vi "ProgramControl.vi"(0 "Universal Robot.lvclass in":refnum<class "Universal Robot.lvclass">, 5 "error in (no error)":errorcluster) -> (14 "Universal Robot.lvclass out":refnum<class "Universal Robot.lvclass">, 15 "programReturnStatus":T1, 19 "error out":errorcluster)   [LabVIEW 2016, in "Universal Robot.lvclass"]
uses:
  Universal Robot.lvclass
  ProgramReturnStatus.ctl
  ProgramState.ctl
panel:
  in  "rate":i32=1000
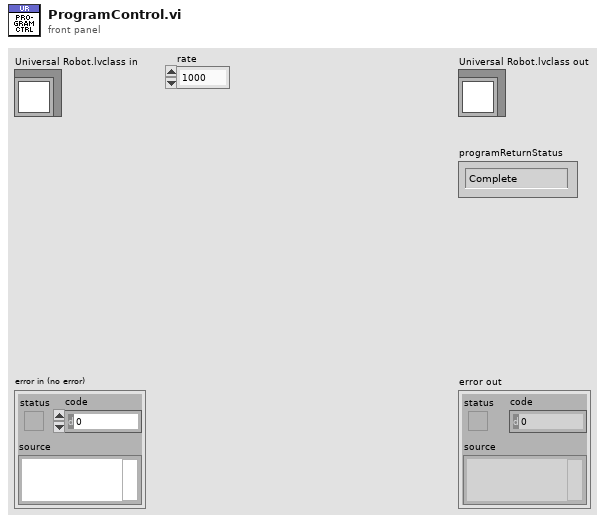
[diagram p1: front panel]
types:
  T1 = typedef "Universal Robot.lvclass/ProgramReturnStatus.ctl" = enum16{"Complete", "Stopped", "Error", "Faulted"}
  T2 = typedef "Universal Robot.lvclass/ProgramState.ctl" = enum16{"STOPPED", "PLAYING", "PAUSE"}
  T3 = typedef "Universal Robot.lvclass/ProgramControlEvent.ctl" = enum16{"Stop", "Pause"}
  T4 = typedef "Universal Robot.lvclass/ProgramStatus.ctl" = cluster{"Loaded Program":string, "Valid Program":bool, "Program State":T2, "Running":bool}
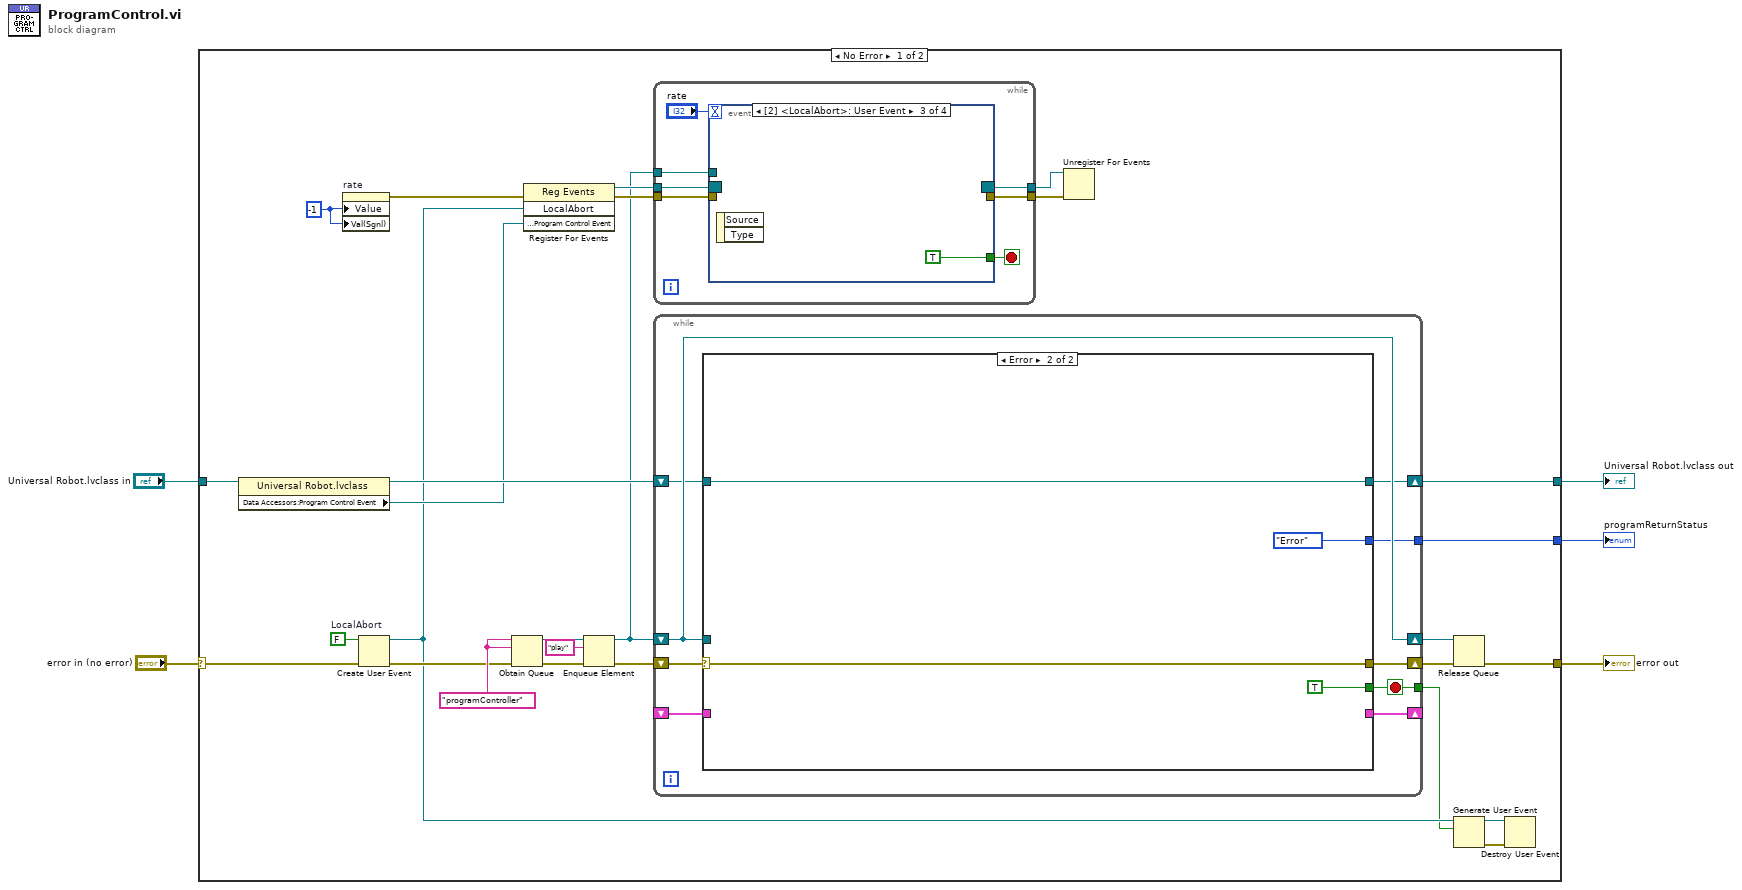
[diagram p0: block diagram]
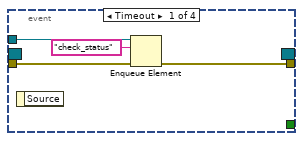
[diagram p2: hidden frame]
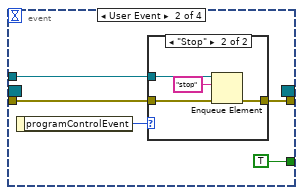
[diagram p3: hidden frame]
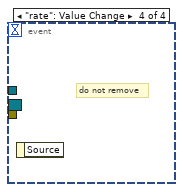
[diagram p5: hidden frame]
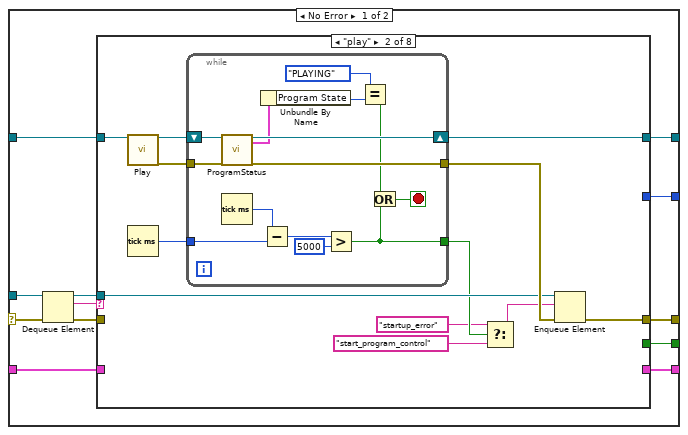
[diagram p6: hidden frame]
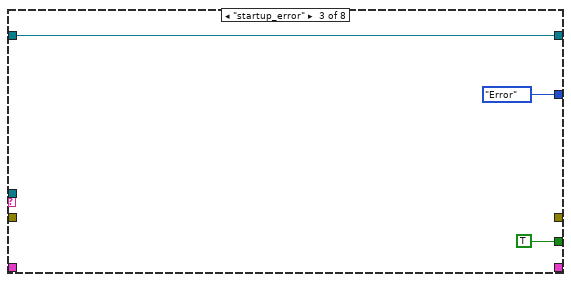
[diagram p8: hidden frame]
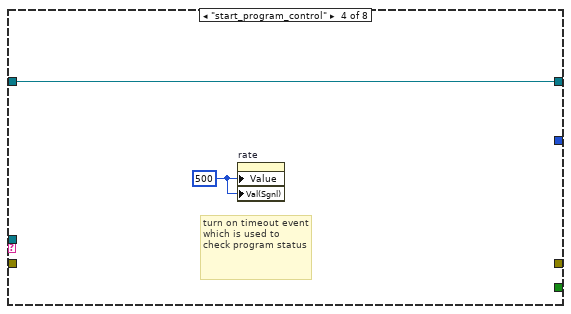
[diagram p9: hidden frame]
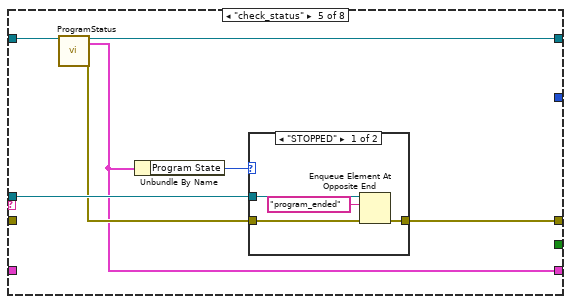
[diagram p10: hidden frame]
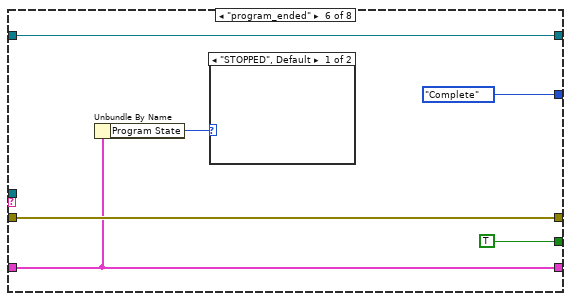
[diagram p12: hidden frame]
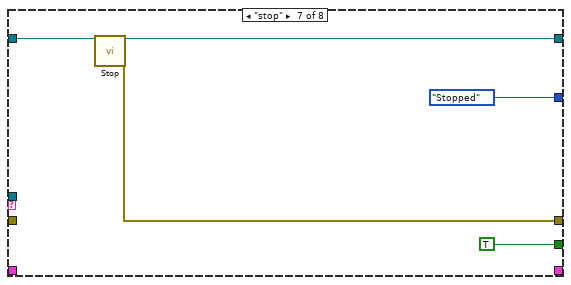
[diagram p14: hidden frame]
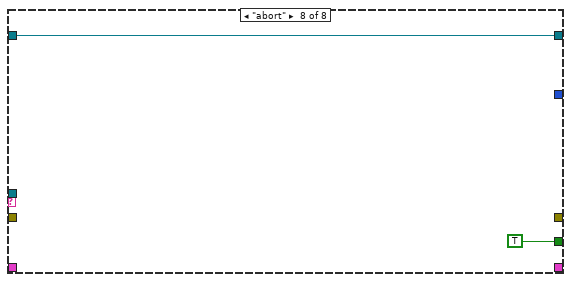
[diagram p15: hidden frame]
diagram:
  n1 = case shown="No Error" "error in (no error)" {
    selector: "error in (no error)" -> [w7 w139]
    tunnel: "Universal Robot.lvclass in" -> [w22 w138]
    tunnel: [w19 _] -> w4
    tunnel: [w9 w139] -> w3
    tunnel: [w8 w138] -> w2
    frame No Error {
      w18 = FALSE  # LocalAbort
      w21 = -1 ("rate")
      w28 = "programController" ("name (unnamed)")
      n2 = property class="Universal Robot.lvclass"(reference=w22) -> (reference out=w27:refnum<class "Universal Robot.lvclass">, "Data Accessors:Program Control Event"=w20:refnum<user-event>)  [unwired: 1 in, 1 out]
      n3 = property on="rate" class="DigNum (strict)"("Value"=w21, "Val(Sgnl)"=w21) -> (error out=w17:errorcluster)  [unwired: 2 in, 1 out]
      n4 = Create User Event(user event datatype=w18, error in=w7) -> (user event=w14:refnum<user-event>, error out=w16:errorcluster)
      n5 = Obtain Queue(name (unnamed)=w28, element data type=w28, error in (no error)=w16) -> (queue out=w26:refnum<queue>, error out=w25:errorcluster)  [unwired: 2 in, 1 out]
      n6 = register-events(error in=w17, w14, w20) -> (reference out=w32:refnum<event-registration>, error out=w31:errorcluster)  [unwired: 1 in]
      n7 = Enqueue Element(queue=w26, element="play", error in (no error)=w25) -> (queue out=w24:refnum<queue>, error out=w23:errorcluster)  [unwired: 1 in, 1 out]
      n8 = while {
        tunnel: w24 -> [w39]
        tunnel: w31 -> [w38]
        tunnel: w32 -> [w37]
        tunnel: [w36] -> w10
        tunnel: [w33] -> w11
        stop <- w35 stop-if-true
        n9 = event shown="[2] <LocalAbort>: User Event" {
          selector: w37 -> [_ _ _ _]
          dyn-events: [_ _ _ _] -> w33
          timeout: "rate" -> [_ _ _ _]
          tunnel: w39 -> [w43 w48 _ _]
          tunnel: w38 -> [w42 w47 _ _]
          tunnel: [w41 w46 _ _] -> w36
          tunnel: [_ TRUE TRUE _] -> w35
          event Timeout {
            n10 = event-data() -> ()  [unwired: 1 in, 1 out]
            n11 = Enqueue Element(queue=w43, element="check_status", error in (no error)=w42) -> (error out=w41:errorcluster)  [unwired: 1 in, 2 out]
          }
          event User Event {
            n12 = event-data() -> ("programControlEvent"=w44:T3)  [unwired: 1 in]
            n13 = case shown="\"Stop\"" w44 {
              tunnel: w48 -> [_ w53]
              tunnel: w47 -> [w49 w52]
              tunnel: [w49 w51] -> w46
              frame Default {
              }
              frame "Stop" {
                n14 = Enqueue Element(queue=w53, element="stop", error in (no error)=w52) -> (error out=w51:errorcluster)  [unwired: 1 in, 2 out]
              }
            }
          }
          event User Event {
            n15 = event-data() -> ()  [unwired: 1 in, 2 out]
          }
          event "rate": Value Change {
            # "do not remove"
            n16 = event-data() -> ()  [unwired: 1 in, 1 out]
          }
        }
      }
      n17 = while {
        shift-right: [w61] -> w30
        shift-left: w23 -> [w63]
        shift-right: [w62] -> w29
        shift-left: w24 -> [w62]
        shift-right: [w59] -> w8
        shift-left: w27 -> [w60]
        shift-right: [w58] -> _
        shift-left: _ -> [w57]
        tunnel: [w56] -> w19
        tunnel: [w55] -> w6
        stop <- w55 stop-if-true
        n18 = case shown="Error" w63 {
          selector: w63 -> [w74 w135]
          tunnel: w62 -> [w75 _]
          tunnel: [w70 w135] -> w61
          tunnel: [w69 TRUE] -> w55
          tunnel: w60 -> [w68 w137]
          tunnel: [w67 w137] -> w59
          tunnel: [w66 _] -> w58
          tunnel: w57 -> [w65 _]
          tunnel: [w64 ProgramReturnStatus."Error" ("programReturnStatus")] -> w56
          frame No Error {
            n19 = Dequeue Element(queue=w75, error in (no error)=w74) -> (queue out=w71:refnum<queue>, element=w72:string, error out=w73:errorcluster)  [unwired: 1 in, 1 out]
            n20 = case shown="\"play\"" w72 {
              tunnel: w73 -> [w77 _ _ _ _ w125 _ _]
              tunnel: w71 -> [_ w82 _ _ w113 _ _ _]
              tunnel: [w77 w84 _ _ w111 w125 w127 _] -> w70
              tunnel: [_ _ TRUE _ _ TRUE TRUE TRUE] -> w69
              tunnel: w68 -> [w76 w89 w106 w108 w115 w126 w129 w132]
              tunnel: [w76 w87 w106 w108 w114 w126 w128 w132] -> w67
              tunnel: [_ _ _ _ w110 w123 _ _] -> w66
              tunnel: w65 -> [_ _ _ _ _ w123 _ _]
              tunnel: [_ _ ProgramReturnStatus."Error" ("programReturnStatus") _ _ ProgramReturnStatus."Complete" ("programReturnStatus") ProgramReturnStatus."Stopped" ("programReturnStatus") _] -> w64
              frame Default {
              }
              frame "play" {
                n21 = call-dynamic "Play.vi"("Universal Robot.lvclass in"=w89) -> ("Universal Robot.lvclass out"=w88:refnum<class "Universal Robot.lvclass">, "error out"=w86:errorcluster)  [unwired: 17 in]
                n22 = Tick Count (ms)() -> (millisecond timer value=w85:u32)
                n23 = while {
                  shift-right: [w102] -> w87
                  shift-left: w88 -> [w103]
                  tunnel: w86 -> [w100]
                  tunnel: w85 -> [w98]
                  tunnel: [w97] -> w83
                  tunnel: [w93] -> w81
                  stop <- w94 stop-if-true
                  n24 = call-dynamic "ProgramStatus.vi"("Universal Robot.lvclass in"=w103, "error in (no error)"=w100) -> ("Universal Robot.lvclass out"=w102:refnum<class "Universal Robot.lvclass">, "Program Status"=w101:T4, "error out"=w97:errorcluster)  [unwired: 15 in]
                  n25 = Tick Count (ms)() -> (millisecond timer value=w99:u32)
                  n26 = Unbundle By Name(w101) -> ("Program State"=w92:T2)
                  n27 = Subtract(x=w99, y=w98) -> (x-y=w96:u32)
                  n28 = Greater?(x=w96, y=u32 5000) -> (0:w93:bool)
                  n29 = Equal?(x=ProgramState."PLAYING", y=w92) -> (x = y?=w90:bool)
                  n30 = Or(x=w90, y=w93) -> (x .or. y?=w94:bool)
                }
                n31 = Select(t="startup_error", s=w81, f="start_program_control") -> (s? t:f=w79:string)
                n32 = Enqueue Element(queue=w82, element=w79, error in (no error)=w83) -> (error out=w84:errorcluster)  [unwired: 1 in, 2 out]
              }
              frame "startup_error" {
              }
              frame "start_program_control" {
                w107 = 500 ("rate")
                # "turn on timeout event which is used to check program status"
                n33 = property on="rate" class="DigNum (strict)"("Value"=w107, "Val(Sgnl)"=w107) -> ()  [unwired: 2 in, 2 out]
              }
              frame "check_status" {
                n34 = call-dynamic "ProgramStatus.vi"("Universal Robot.lvclass in"=w115) -> ("Universal Robot.lvclass out"=w114:refnum<class "Universal Robot.lvclass">, "Program Status"=w110:T4, "error out"=w112:errorcluster)  [unwired: 16 in]
                n35 = Unbundle By Name(w110) -> ("Program State"=w109:T2)
                n36 = case shown="\"STOPPED\"" w109 {
                  tunnel: w113 -> [w119 _]
                  tunnel: w112 -> [w118 w120]
                  tunnel: [w117 w120] -> w111
                  frame "STOPPED" {
                    n37 = Enqueue Element At Opposite End(queue=w119, element="program_ended", error in (no error)=w118) -> (error out=w117:errorcluster)  [unwired: 1 in, 2 out]
                  }
                  frame Default {
                  }
                }
              }
              frame "program_ended" {
                n38 = Unbundle By Name(w123) -> ("Program State"=w122:T2)
                n39 = case shown="\"STOPPED\", Default" w122 {
                  frame "STOPPED", Default {
                  }
                  frame "PLAYING" {
                  }
                }
              }
              frame "stop" {
                n40 = call-dynamic "Stop.vi"("Universal Robot.lvclass in"=w129) -> ("Universal Robot.lvclass out"=w128:refnum<class "Universal Robot.lvclass">, "error out"=w127:errorcluster)  [unwired: 17 in]
              }
              frame "abort" {
              }
            }
          }
          frame Error {
          }
        }
      }
      n41 = Unregister For Events(event registration refnum=w11, error in=w10) -> ()  [unwired: 1 out]
      n42 = Release Queue(queue=w29, error in (no error)=w30) -> (error out=w9:errorcluster)  [unwired: 1 in, 2 out]
      n43 = Generate User Event(user event=w14, event data cluster=w6) -> (user event out=w13:refnum<user-event>, error out=w12:errorcluster)  [unwired: 2 in]
      n44 = Destroy User Event(user event=w13, error in=w12) -> ()  [unwired: 1 out]
    }
    frame Error {
    }
  }
  "error out" <- w3
  "Universal Robot.lvclass out" <- w2
  "programReturnStatus" <- w4
